vi "Type Panel.vi"(11 "IntegerPanel in":refnum<class "IntegerPanel.lvclass">) -> ()   [LabVIEW 2020, in "Conditum-Tools.lvlib" / "IntegerPanel.lvclass"]
uses:
  IntegerPanel.lvclass
panel:
  in  "Default":i64
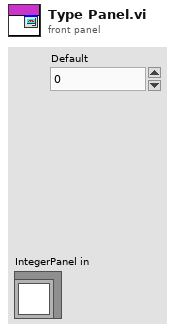
[diagram p1: front panel]
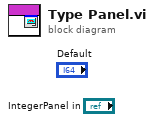
[diagram p0: block diagram]
diagram:
